vi "Create Chans.vi"(5 "New Section Name (none)":string, 7 "Type":T2=enum."Output", 8 "error in (no error)":errorcluster, 10 "Channels":T1[](array[typedef]), 11 "Section Ptr":T3 format="%.0x") -> (0 "error out":errorcluster, 3 "Section Ptr dup":T3 format="%.0x")   [LabVIEW 2017, in "PXImc System Explorer.lvlib"]
uses:
  PXImc System Explorer.lvlib
  <vilib>/NI Veristand/Custom Device API/Custom Device Item Ref.ctl
  <vilib>/NI Veristand/Custom Device API/Custom Device Channel Type.ctl
  Shared/Channel.ctl
  Shared/Constants.vi
  <vilib>/NI VeriStand/Custom Device API/Custom Device API.lvlib
  Shared/PXImc Shared.lvlib
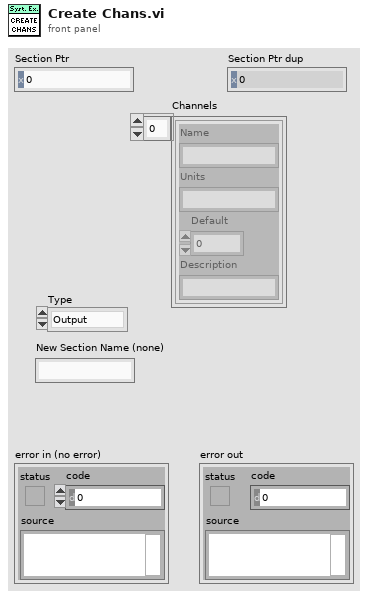
[diagram p1: front panel]
types:
  T1 = typedef "PXImc Shared.lvlib/Channel.ctl" = cluster{"Name":string, "Units":string, "Default":dbl, "Description":string}
  T2 = typedef "Custom Device API.lvlib/Custom Device Channel Type.ctl" = enum16{"Input", "Output"}
  T3 = typedef "Custom Device API.lvlib/Custom Device Item Ref.ctl" = u64
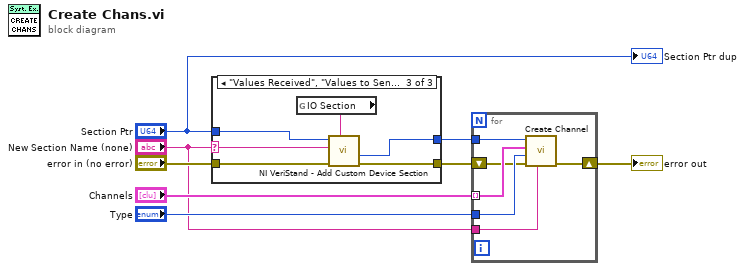
[diagram p0: block diagram]
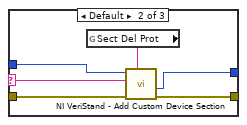
[diagram p3: hidden frame]
diagram:
  n1 = case shown="\"Values Received\", \"Values to Send\"" "New Section Name (none)" {
    selector: "New Section Name (none)" -> [_ w12 w18]
    tunnel: "error in (no error)" -> [w10 w16 w22]
    tunnel: "Section Ptr" -> [w9 w15 w21]
    tunnel: [w10 w14 w20] -> w5
    tunnel: [w9 w13 w19] -> w4
    frame "" {
    }
    frame Default {
      n2 = global read "Constants.vi" "Sect Del Prot"() -> (w11:string)
      n3 = call <vilib>:"NI VeriStand - Add Custom Device Section.vi"("GUID (Default Section)"=w11, "error in (no error)"=w16, "Section Name"=w12, "Parent Ref in"=w15) -> ("error out"=w14:errorcluster, "Section Ptr"=w13:T3)  [unwired: 4 in, 2 out]
    }
    frame "Values Received", "Values to Send" {
      n4 = global read "Constants.vi" "IO Section"() -> (w17:string)
      n5 = call <vilib>:"NI VeriStand - Add Custom Device Section.vi"("GUID (Default Section)"=w17, "error in (no error)"=w22, "Section Name"=w18, "Parent Ref in"=w21) -> ("error out"=w20:errorcluster, "Section Ptr"=w19:T3)  [unwired: 4 in, 2 out]
    }
  }
  n6 = for {
    tunnel: w4 -> [w28]
    shift-right: [w24] -> w7
    shift-left: w5 -> [w25]
    tunnel: "Channels" -> [w26] mode=indexing
    tunnel: "Type" -> [w27]
    tunnel: "New Section Name (none)" -> [w23]
    n7 = call "Create Channel.vi"("New Section Name (none)"=w23, "error in"=w25, "Type"=w27, "Channel"=w26, "Item Ref in"=w28) -> ("error out"=w24:errorcluster)  [unwired: 5 in, 1 out]
  }
  "error out" <- w7
  "Section Ptr dup" <- "Section Ptr"
